vi "example_one.vi"() -> ()   [LabVIEW 2012]
uses:
  <vilib>/ptbypt/NI_PtbyPt.lvlib
panel:
  out "Waveform Chart 3":i32(graph)
  out "Waveform Chart 2":dbl(graph)
  out "Waveform Chart":dbl(graph)
  out ".not. x?":bool
  in  "stop":bool
  out "Meter":dbl(knob) scale=0.0..100.0
  out "x > y?":bool
  out "x*y":dbl
  in  "Slide 2":dbl(slide) scale=0.0..10.0
  in  "Slide":dbl(slide) scale=0.0..10.0
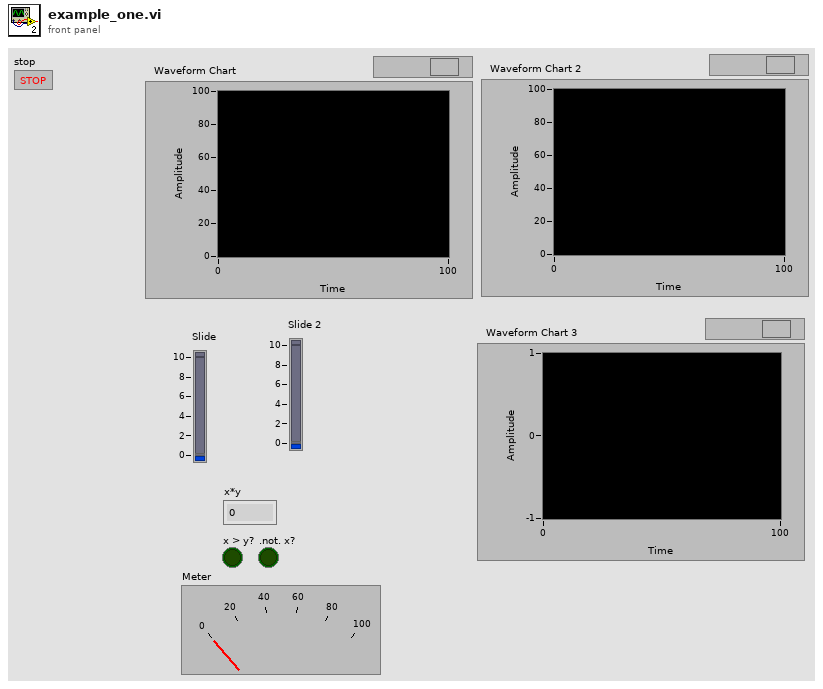
[diagram p1: front panel]
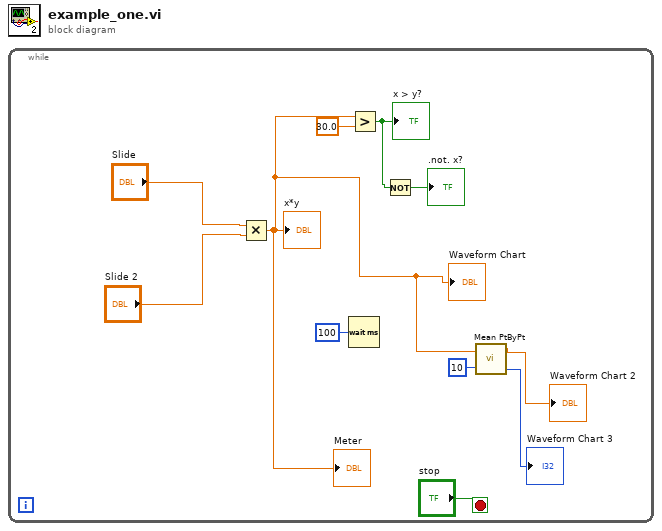
[diagram p0: block diagram]
diagram:
  n1 = while {
    stop <- "stop" stop-if-true
    n2 = Multiply(x="Slide", y="Slide 2") -> (x*y=w4:dbl)
    "x*y" <- w4
    "Meter" <- w4
    "Waveform Chart" <- w4
    n3 = Wait (ms)(milliseconds to wait=u32 100) -> ()  [unwired: 1 out]
    n4 = Greater?(x=w4, y=30.0) -> (0:w7:bool)
    "x > y?" <- w7
    n5 = Not(x=w7) -> (.not. x?=→".not. x?":bool)
    n6 = call <vilib>:"Mean PtByPt.vi"("x"=w4, "sample length"=10) -> ("mean"=→"Waveform Chart 2":dbl, "error"=→"Waveform Chart 3":i32)  [unwired: 2 in]
  }
